vi "LiDARSteering.vi"() -> ()   [LabVIEW 2024]
uses:
  e33ea129-5426-40bd-9da2-e127971607b1.vi
  <vilib>/Instr/_visa.llb/VISA Configure Serial Port (Instr).vi
  <vilib>/Python/Open Venv Python Session.vi
  <vilib>/Instr/_visa.llb/VISA Set IO Buffer Mask.ctl
  <vilib>/Instr/_visa.llb/VISA Flush IO Buffer Mask.ctl
panel:
  out "inputsteer":dbl format="%#_13g"
  in  "HENES":refnum<visa-resource-name>="COM3"
  out "E-STOP":bool
  out "Remote_M/A":bool
  out "Steer_Feed":dbl
  out "Alive_PCU":u8(slide) scale=0.0..254.0
  out "Gear_Feed":u8
  out "Speed_Feed(RPM)":dbl format="%#_g rpm"
  out "버퍼 읽기":string
  out "Speed_Feed(m/s)":dbl
  in  "HLV_Gear 2":u8
  in  "HLV_A/M":bool=TRUE
  in  "HLV_E-stop":bool
  out "버퍼 쓰기":string
  in  "InputSpeed":i16
  out "HENES Loop Time":u32=20
  out "Input_Spd(cmd)":dbl=538.4742241275792
  in  "GoBack":bool
  in  "InputSteer(cmd)":dbl=28.559259641865033
  in  "HLV_Gear":u8
  out "PointCloud":T1(graph)=[{"appended array"=[700.0, 700.0, 3500.0, 3500.0, -3500.0, -3500.0, -700.0, -700.0, 700.0], "appended array"=[800.0, -800.0, -800.0, 5200.0, 5200.0, -800.0, -800.0, 800.0, 800.0]}, {"appended array"=[-450.0], "appended array"=[-250.0]}, {"appended array"=[-450.0, -450.0, -800.0, -800.0, 0.0, 0.0, -450.0], "appended array"=[100.0, -800.0, -800.0, 1200.0, 1200.0, 100.0, 100.0]}, {"appended array"=[800.0, 750.0, 800.0, 800.0, 800.0, 800.0, 800.0], "appended array"=[400.0, 350.0, 350.0, 300.0, 250.0, 200.0, 150.0]}, {"appended array"=[450.0, 450.0, 800.0, 800.0, 0.0, 0.0, 450.0], "appended array"=[100.0, -800.0, -800.0, 1200.0, 1200.0, 100.0, 100.0]}, {"appended array"=array[442 elements], "appended array"=array[442 elements]}, {"appended array"=[4.2861222383783204e-13, 0.0], "appended array"=[7000.0, 0.0]}, {"appended array"=[500.0, 500.0, -500.0, -500.0, 500.0], "appended array"=[100.0, 950.0, 950.0, 100.0, 100.0]}]
  in  "격자크기":dbl=50.0
  out "LidarLoop":u32=101
  in  "Ratio_Threshold":i32=4
  in  "min_samples":i32=2
  in  "eps":i32=100
  in  "Spacing":i32=100
  in  "Threshold":i32=2100
  in  "Looking Y":i32=5200
  in  "Looking X":i32=3500
  out "Anthena_Steer":i32
  out "NearSteer":dbl=28.559259641865033
  out "TooClose":bool=TRUE
  out "PythonLoop":u32=101
  in  "LiDAR":refnum<visa-resource-name>="COM5"
  out "VEstop":bool
  in  "length":dbl=1300.0
  out "read buffer":string
  out "Clustering Error":errorcluster
  out "GobackROI":cluster{i32[], i32[]}={[500, 500, -500, -500, 500], [100, 950, 950, 100, 100]}
  in  "Stop":bool
  out "TargetDerection":cluster{dbl[], dbl[]}={[4.2861222383783204e-13, 0.0], [7000.0, 0.0]}
  out "Y_arraysREAL":i32[](array[numeric])=[1650, 1650, 1650, 1650, 1650, 1650, 1650, 1650, 1700, 1700, 1700, 1700, 1700, 1700, 1700, 1700, 1700, 1700, 1700, 1750, 1700]
  out "X_arraysREAL":i32[](array[numeric])=[1000, 1050, 1100, 1150, 1200, 1250, 1300, 1350, 1350, 1400, 1450, 1500, 1550, 1600, 1650, 1700, 1750, 1800, 1850, 1850, 1900]
  out "LookingAt":cluster{i32[], i32[]}={[700, 700, 3500, 3500, -3500, -3500, -700, -700, 700], [800, -800, -800, 5200, 5200, -800, -800, 800, 800]}
  out "NearCarPointsRight":cluster{"ROI_IN_X":dbl[], "ROI_IN_Y":dbl[]}={"ROI_IN_X"=[750.0, 800.0, 800.0, 800.0, 800.0, 800.0], "ROI_IN_Y"=[350.0, 350.0, 300.0, 250.0, 200.0, 150.0]}
  out "NearCarROIRight":cluster{i32[], i32[]}={[450, 450, 800, 800, 0, 0, 450], [100, -800, -800, 1200, 1200, 100, 100]}
  out "Clustered":T2
  out "NearCarROILeft":cluster{i32[], i32[]}={[-450, -450, -800, -800, 0, 0, -450], [100, -800, -800, 1200, 1200, 100, 100]}
  out "NearCarPointsLeft":cluster{"ROI_IN_X":dbl[], "ROI_IN_Y":dbl[]}={"ROI_IN_X"=[-450.0, -550.0], "ROI_IN_Y"=[-250.0, -300.0]}
  out "Y_arrays":dbl[](array[numeric])=[1650.0, 1650.0, 1650.0, 1650.0, 1650.0, 1650.0, 1650.0, 1700.0, 1700.0, 1700.0, 1700.0, 1700.0, 1700.0, 1700.0, 1700.0, 1700.0, 1700.0, 1700.0, 1750.0, 1700.0, 1700.0, 1750.0, 1750.0, 1750.0, 1750.0, 1750.0, 1750.0, 1750.0, 1750.0, 1750.0, 1750.0, 1750.0, 1800.0, 1800.0, 1800.0, 1800.0, 1800.0, 1800.0, 1800.0, 1800.0, 1800.0, 1800.0, 1800.0, 1800.0, 1800.0, 1800.0, 1800.0, 1800.0, 1800.0, 1850.0, 1850.0, 1850.0, 350.0, 350.0, 350.0, 300.0, 250.0, 200.0, 200.0, 150.0, 150.0, 100.0, 50.0, 0.0, -50.0, -100.0, -150.0, -200.0, -250.0, -300.0, -300.0, -350.0, -400.0, -450.0, -500.0, -550.0, -600.0, -650.0, -700.0, -750.0, -800.0, -800.0, -750.0, -750.0, -700.0, -700.0, -650.0, -600.0, -550.0, -550.0, -500.0, -450.0, -400.0, -350.0, -300.0, -250.0, -200.0, -150.0, -100.0, -50.0, 0.0, 50.0, 100.0, 150.0, 200.0, 250.0, 300.0, 350.0, 400.0, 400.0, 450.0, 500.0, 550.0, 600.0, 600.0, 650.0, 650.0, 700.0, 700.0, 750.0, 750.0, 800.0, 800.0, 850.0, 850.0, 900.0, 900.0, 950.0, 950.0, 1000.0, 1000.0, 1050.0, 1050.0, 1100.0, 1100.0, 1150.0, 1150.0, 1200.0, 1200.0, 1250.0, 1250.0, 1300.0, 1300.0, 1350.0, 1400.0, 1450.0, 1500.0, 1550.0, 1600.0, 1650.0, 1700.0, 1750.0, 1800.0, 1850.0, 1900.0, 1950.0, 2000.0, 2050.0, 2100.0, 2150.0, 2200.0, 2250.0, 2300.0, 2350.0, 2400.0, 2450.0, 2500.0, 2550.0, 2600.0, 2600.0, 2650.0, 2700.0, 2750.0, 2800.0, 2850.0, 2900.0, 2950.0, 3000.0, 3050.0, 3100.0, 3150.0, 3200.0, 3250.0, 3300.0, 3350.0, 3400.0, 3450.0, 3450.0, 3500.0, 3550.0, 3600.0, 3650.0, 3700.0, 3750.0, 3800.0, 3850.0, 3900.0, 3950.0, 4000.0, 4000.0, 4100.0, 4150.0, 4200.0, 4250.0, 4300.0, 4350.0, 4400.0, 4450.0, 4500.0, 4550.0, 4600.0, 4650.0, 4700.0, 4750.0, 4800.0, 4900.0, 4950.0, 5000.0, 5050.0, 5100.0, 5150.0, 4500.0, 4500.0, 4600.0, 4550.0, 3800.0, 3700.0, 3650.0, 3600.0, 3550.0, 3500.0, 3500.0, 3450.0, 3400.0, 3350.0, 3300.0, 3250.0, 3250.0, 3200.0, 3150.0, 3200.0, 3200.0, 3200.0, 3400.0, 3450.0, 3200.0, 4700.0, 4700.0, 3700.0, 3450.0, 3400.0, 3450.0, 3500.0, 3500.0, 3450.0, 3400.0, 3400.0, 3350.0, 3300.0, 3300.0, 3250.0, 1600.0, 1600.0, 1650.0, 1600.0, 1650.0, 1735.0877192982457, -160.3448275862069, 1825.7462686567164, 5025.0, 4500.0, 4575.0, 3392.1052631578946, 3425.0, 4700.0, 3395.8333333333335, 1827.3513645224173, 1919.6150097465888, 2011.8786549707602, 2104.142300194932, 2196.4059454191033, 2288.669590643275, 2380.9332358674465, 2473.196881091618, 2565.4605263157896, 2657.7241715399614, 2749.9878167641327, 2842.251461988304, 2934.5151072124754, 3026.778752436647, 3119.042397660819, 3211.3060428849903, 3303.5696881091617, 1824.0304709141276, 1912.9732225300093, 2001.9159741458911, 2090.858725761773, 2179.801477377655, 2268.7442289935366, 2357.6869806094182, 2446.6297322253004, 2535.572483841182, 2624.5152354570637, 2713.457987072946, 2802.400738688827, 2891.343490304709, 2980.2862419205912, 3069.228993536473, 3158.1717451523546, 3247.114496768236, 3336.057248384118, 1817.938596491228, 1900.7894736842106, 1983.640350877193, 2066.4912280701756, 2149.342105263158, 2232.1929824561403, 2315.043859649123, 2397.8947368421054, 2480.745614035088, 2563.59649122807, 2646.4473684210525, 2729.2982456140353, 2812.149122807017, 2895.0, 2977.8508771929824, 3060.7017543859647, 3143.5526315789475, 3226.4035087719294, 3309.254385964912, 4515.0, 4530.0, 4545.0, 4560.0, 4407.675438596491, 4315.350877192983, 4223.026315789473, 4130.701754385965, 4038.377192982456, 3946.0526315789475, 3853.7280701754385, 3761.40350877193, 3669.078947368421, 3576.754385964912, 3484.4298245614036, 4417.307692307692, 4334.615384615385, 4251.923076923077, 4169.2307692307695, 4086.5384615384614, 4003.846153846154, 3921.153846153846, 3838.4615384615386, 3755.769230769231, 3673.076923076923, 3590.3846153846152, 3507.6923076923076, 4588.888888888889, 4602.777777777777, 4616.666666666667, 4630.555555555556, 4644.444444444444, 4658.333333333333, 4672.222222222223, 4686.111111111111, 4479.166666666667, 4383.333333333333, 4287.5, 4191.666666666667, 4095.8333333333335, 4000.0, 3904.166666666667, 3808.3333333333335, 3712.5, 3616.666666666667, 3520.8333333333335, 3403.0701754385964, 3414.035087719298, 3392.6378446115286, 3393.1704260651627, 3393.7030075187968, 3394.2355889724313, 3394.7681704260654, 3395.3007518796994, 3417.7083333333335, 3410.416666666667, 3403.125, 4684.615384615385, 4669.2307692307695, 4653.846153846154, 4638.461538461538, 4623.076923076923, 4607.692307692308, 4592.307692307692, 4576.923076923077, 4561.538461538462, 4546.153846153846, 4530.7692307692305, 4515.384615384615, 4606.8452380952385, 4513.690476190476, 4420.535714285715, 4327.380952380952, 4234.226190476191, 4141.071428571428, 4047.916666666667, 3954.761904761905, 3861.607142857143, 3768.452380952381, 3675.2976190476193, 3582.1428571428573, 3488.9880952380954, 3486.538461538462, 3577.24358974359, 3667.9487179487182, 3758.653846153846, 3849.3589743589746, 3940.0641025641025, 4030.769230769231, 4121.474358974359, 4212.179487179487, 4302.884615384615, 4393.589743589744, 4484.294871794872]
  out "X_arrays":dbl[](array[numeric])=[1050.0, 1100.0, 1150.0, 1200.0, 1250.0, 1300.0, 1350.0, 1350.0, 1400.0, 1450.0, 1500.0, 1550.0, 1600.0, 1650.0, 1700.0, 1750.0, 1800.0, 1850.0, 1850.0, 1900.0, 1950.0, 2000.0, 2050.0, 2100.0, 2150.0, 2200.0, 2250.0, 2300.0, 2350.0, 2400.0, 2450.0, 2500.0, 2500.0, 2550.0, 2600.0, 2650.0, 2700.0, 2750.0, 2800.0, 2850.0, 2900.0, 2950.0, 3000.0, 3050.0, 3100.0, 3150.0, 3200.0, 3250.0, 3300.0, 3350.0, 3400.0, 3450.0, 750.0, 800.0, 850.0, 800.0, 800.0, 800.0, 850.0, 800.0, 850.0, 850.0, 850.0, 850.0, 850.0, 850.0, 850.0, 850.0, 850.0, 850.0, 900.0, 900.0, 900.0, 900.0, 900.0, 900.0, 900.0, 900.0, 900.0, 900.0, 900.0, -2250.0, -2250.0, -2300.0, -2300.0, -2250.0, -2300.0, -2300.0, -2300.0, -2350.0, -2300.0, -2300.0, -2300.0, -2300.0, -2300.0, -2300.0, -2300.0, -2300.0, -2300.0, -2300.0, -2300.0, -2300.0, -2300.0, -2300.0, -2300.0, -2300.0, -2300.0, -2300.0, -2250.0, -2300.0, -2300.0, -2300.0, -2300.0, -2300.0, -2250.0, -2250.0, -2300.0, -2250.0, -2300.0, -2300.0, -2250.0, -2300.0, -2250.0, -2300.0, -2250.0, -2300.0, -2250.0, -2250.0, -2300.0, -2300.0, -2250.0, -2250.0, -2300.0, -2250.0, -2300.0, -2250.0, -2300.0, -2250.0, -2300.0, -2300.0, -2250.0, -2300.0, -2250.0, -2250.0, -2250.0, -2250.0, -2250.0, -2250.0, -2250.0, -2250.0, -2250.0, -2250.0, -2250.0, -2250.0, -2250.0, -2250.0, -2250.0, -2250.0, -2250.0, -2250.0, -2250.0, -2250.0, -2250.0, -2250.0, -2250.0, -2250.0, -2250.0, -2250.0, -2250.0, -2300.0, -2300.0, -2300.0, -2300.0, -2300.0, -2300.0, -2300.0, -2300.0, -2300.0, -2300.0, -2300.0, -2300.0, -2300.0, -2300.0, -2300.0, -2300.0, -2300.0, -2300.0, -2350.0, -2350.0, -2350.0, -2350.0, -2350.0, -2350.0, -2350.0, -2350.0, -2350.0, -2350.0, -2350.0, -2350.0, -2400.0, -2400.0, -2400.0, -2400.0, -2400.0, -2400.0, -2400.0, -2400.0, -2400.0, -2400.0, -2400.0, -2400.0, -2400.0, -2400.0, -2400.0, -2400.0, -2450.0, -2450.0, -2450.0, -2450.0, -2450.0, -2450.0, 650.0, 700.0, 1100.0, 1150.0, 950.0, 950.0, 950.0, 950.0, 950.0, 950.0, 1000.0, 1000.0, 1000.0, 1000.0, 1000.0, 1000.0, 1050.0, 1050.0, 1050.0, 1100.0, 1150.0, 1200.0, 1300.0, 1350.0, 1250.0, 1900.0, 1950.0, 1600.0, 1500.0, 1550.0, 1600.0, 1600.0, 1650.0, 1650.0, 1650.0, 1700.0, 1650.0, 1650.0, 1700.0, 1700.0, 900.0, 950.0, 950.0, 1000.0, 1000.0, 2118.4210526315787, 856.8965517241379, -2300.0, -2450.0, 675.0, 1125.0, 1028.9473684210527, 1325.0, 1925.0, 1633.3333333333333, 2091.4717348927875, 2064.522417153996, 2037.5730994152045, 2010.623781676413, 1983.6744639376216, 1956.7251461988303, 1929.7758284600388, 1902.8265107212474, 1875.877192982456, 1848.9278752436646, 1821.9785575048732, 1795.029239766082, 1768.0799220272904, 1741.130604288499, 1714.1812865497075, 1687.231968810916, 1660.2826510721247, 2076.6620498614957, 2034.9030470914126, 1993.1440443213294, 1951.3850415512463, 1909.6260387811633, 1867.8670360110802, 1826.108033240997, 1784.349030470914, 1742.590027700831, 1700.8310249307478, 1659.0720221606648, 1617.3130193905818, 1575.5540166204987, 1533.7950138504154, 1492.0360110803324, 1450.2770083102494, 1408.5180055401663, 1366.759002770083, 2063.9473684210525, 2009.4736842105262, 1954.9999999999998, 1900.5263157894735, 1846.0526315789473, 1791.5789473684208, 1737.1052631578946, 1682.6315789473683, 1628.157894736842, 1573.6842105263158, 1519.2105263157894, 1464.736842105263, 1410.2631578947367, 1355.7894736842104, 1301.3157894736842, 1246.842105263158, 1192.3684210526317, 1137.8947368421054, 1083.421052631579, 765.0, 855.0, 945.0, 1035.0, 704.4956140350878, 733.9912280701755, 763.4868421052631, 792.9824561403509, 822.4780701754387, 851.9736842105264, 881.469298245614, 910.9649122807018, 940.4605263157896, 969.9561403508773, 999.4517543859649, 725.0, 775.0, 825.0, 875.0, 925.0, 975.0, 1025.0, 1075.0, 1125.0, 1175.0, 1225.0, 1275.0, 1213.888888888889, 1302.7777777777778, 1391.6666666666665, 1480.5555555555557, 1569.4444444444443, 1658.3333333333333, 1747.2222222222222, 1836.111111111111, 1141.6666666666667, 1158.3333333333333, 1175.0, 1191.6666666666667, 1208.3333333333333, 1225.0, 1241.6666666666667, 1258.3333333333333, 1275.0, 1291.6666666666667, 1308.3333333333333, 1127.6315789473686, 1226.3157894736842, 1115.2882205513786, 1201.6290726817042, 1287.96992481203, 1374.310776942356, 1460.6516290726815, 1546.9924812030074, 1402.0833333333333, 1479.1666666666665, 1556.25, 1828.8461538461538, 1732.6923076923076, 1636.5384615384614, 1540.3846153846152, 1444.2307692307693, 1348.076923076923, 1251.9230769230767, 1155.7692307692307, 1059.6153846153848, 963.4615384615385, 867.3076923076922, 771.1538461538462, 1904.1666666666667, 1883.3333333333333, 1862.5, 1841.6666666666667, 1820.8333333333333, 1800.0, 1779.1666666666665, 1758.3333333333333, 1737.5, 1716.6666666666665, 1695.8333333333333, 1675.0, 1654.1666666666665, 1594.230769230769, 1555.128205128205, 1516.0256410256409, 1476.923076923077, 1437.8205128205127, 1398.7179487179487, 1359.6153846153845, 1320.5128205128203, 1281.4102564102564, 1242.3076923076924, 1203.2051282051282, 1164.102564102564]
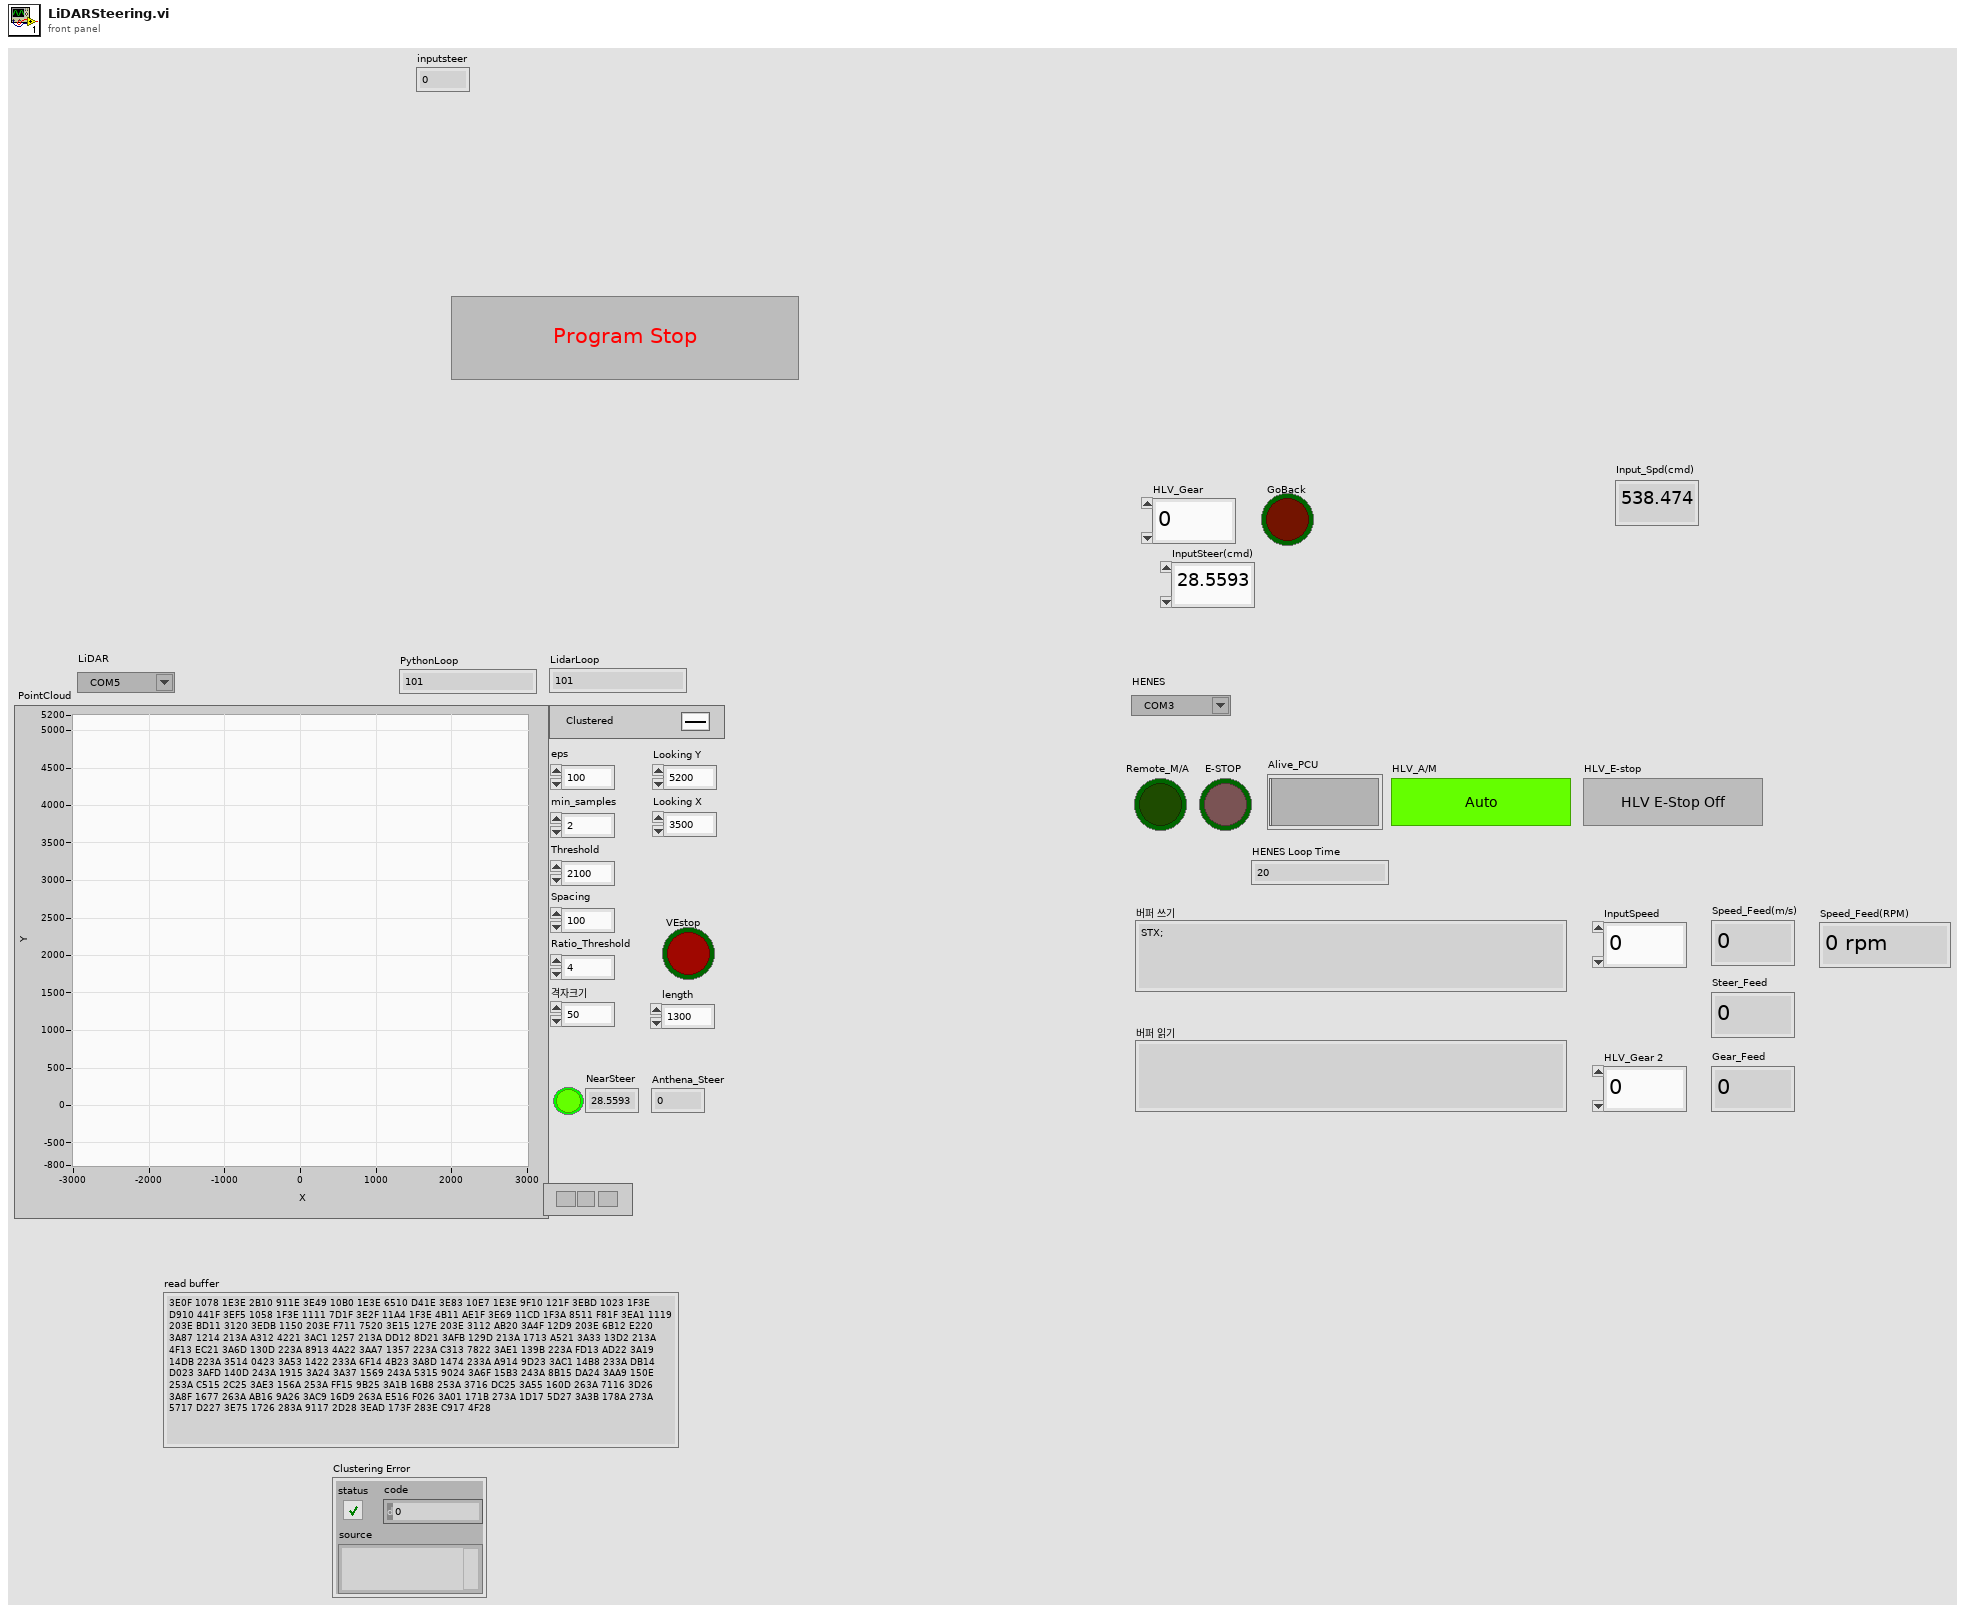
[diagram p1: front panel]
types:
  T1 = cluster{"appended array":dbl[], "appended array":dbl[]}[]
  T2 = cluster{"appended array":dbl[], "appended array":dbl[]}
  T3 = cluster{"HENES_M/A":u8, "HENES_E-Stop":u8, "HENES_Gear":u8, "HENES_Speed":i16, "HENES_Steer":i16, "HENES_Alive":u8}
  T4 = typedef "VISA Flush IO Buffer Mask.ctl" = u16
  T5 = typedef "VISA Set IO Buffer Mask.ctl" = u16
  T6 = cluster{"HLV_M/A_Status":u8, "HLV_E-Stop":u8, "HLV_Gear":u8, "HLV_Speed":i16, "HLV_Steer":i16, "HLV_Alive":u8}
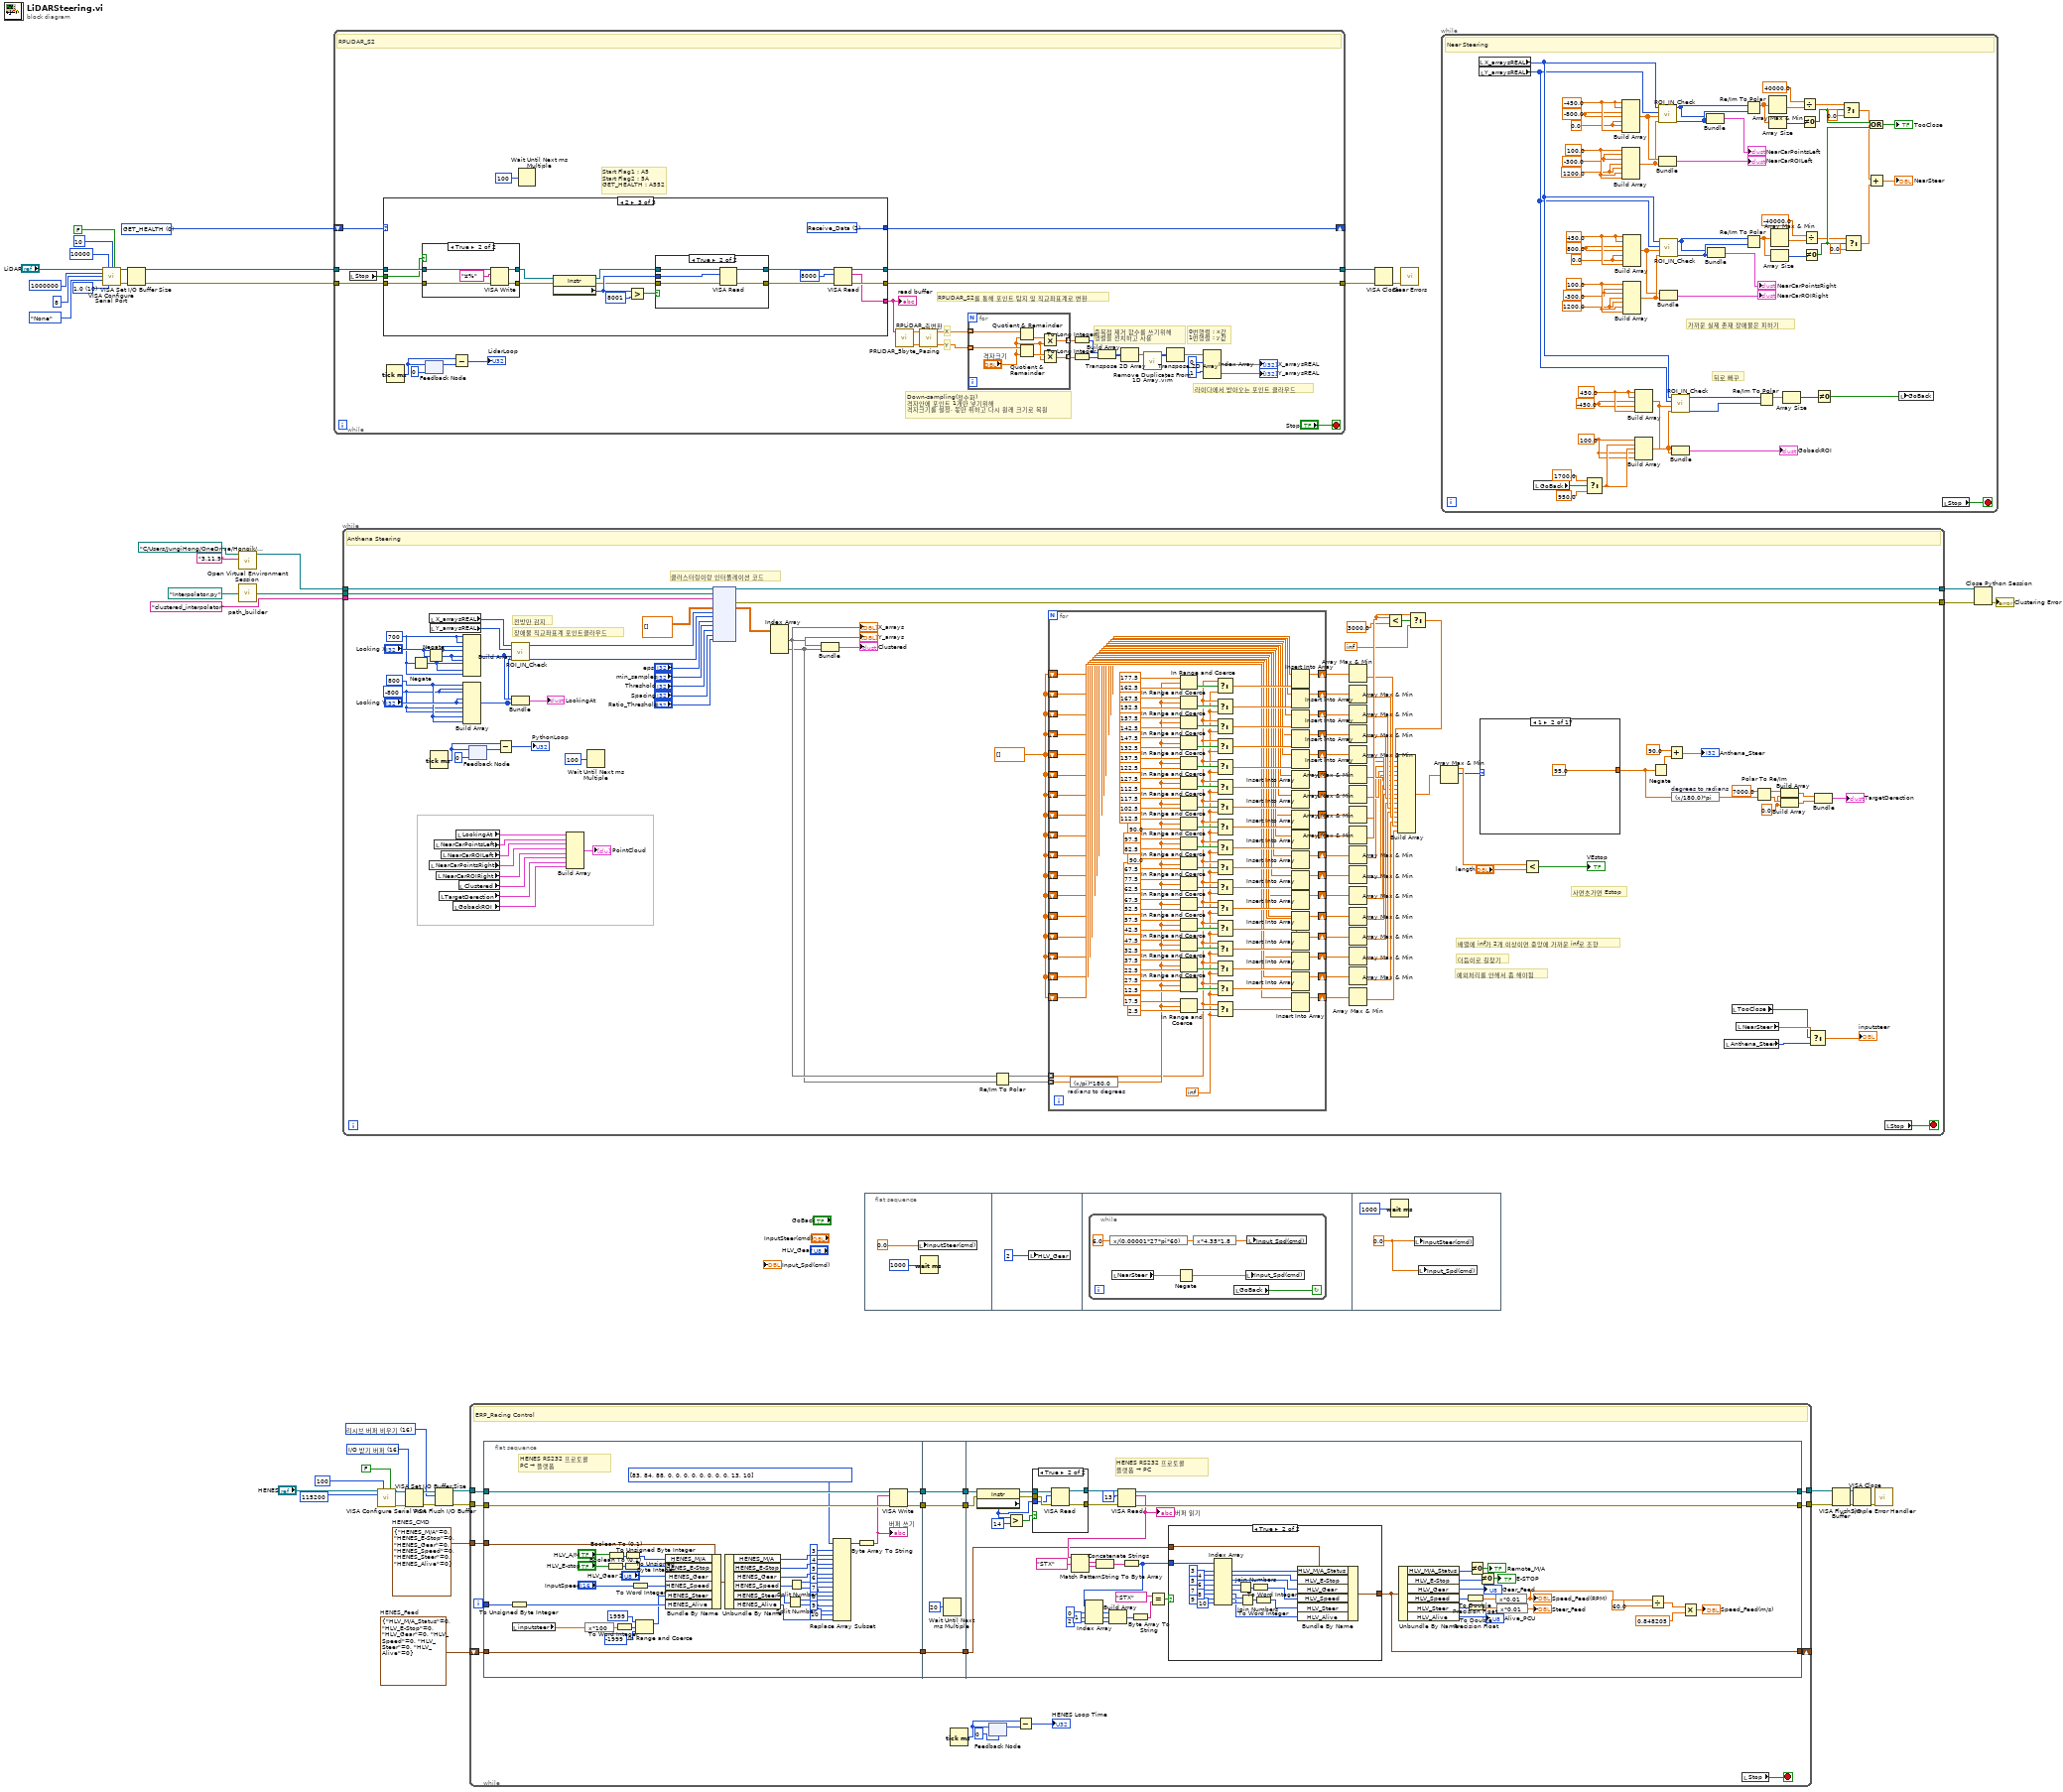
[diagram p0: block diagram]
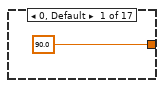
[diagram p4: hidden frame]
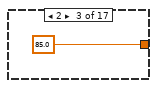
[diagram p5: hidden frame]
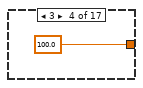
[diagram p6: hidden frame]
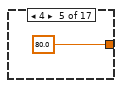
[diagram p7: hidden frame]
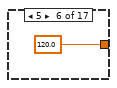
[diagram p8: hidden frame]
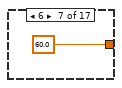
[diagram p9: hidden frame]
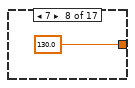
[diagram p10: hidden frame]
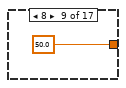
[diagram p11: hidden frame]
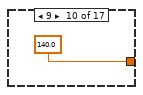
[diagram p12: hidden frame]
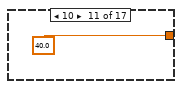
[diagram p13: hidden frame]
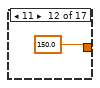
[diagram p14: hidden frame]
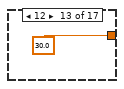
[diagram p15: hidden frame]
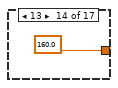
[diagram p16: hidden frame]
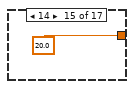
[diagram p17: hidden frame]
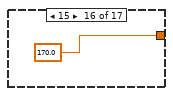
[diagram p18: hidden frame]
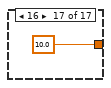
[diagram p19: hidden frame]
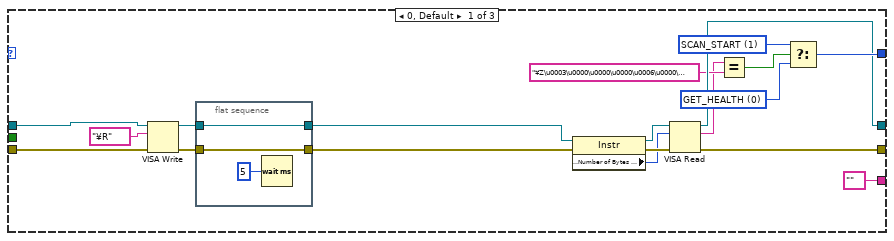
[diagram p20: hidden frame]
diagram:
  w2 = T3 {"HENES_M/A"=0, "HENES_E-Stop"=0, "HENES_Gear"=0, "HENES_Speed"=0, "HENES_Steer"=0, "HENES_Alive"=0}  # HENES_CMD
  w5 = T4 16 items=["리시브 버퍼 비우기"=16, "전달 버퍼 디바이스에 쓰기"=32, "리시브 버퍼 비우기(I/O 없음)"=64, "전달 버퍼 비우기"=128] ("Mask")
  w8 = T5 16 items=["I/O 받기 버퍼"=16, "I/O 전달 버퍼"=32, "I/O 받기와 전달 버퍼"=48] ("Mask")
  w12 = T6 {"HLV_M/A_Status"=0, "HLV_E-Stop"=0, "HLV_Gear"=0, "HLV_Speed"=0, "HLV_Steer"=0, "HLV_Alive"=0}  # HENES_Feed
  w30 = u16 10 items=["1.0"=10, "1.5"=15, "2.0"=20] ("stop bits (10: 1 bit)")
  w32 = u16 0 items=["GET_HEALTH", "SCAN_START", "Receive_Data"]
  n1 = call-poly "VISA Configure Serial Port"("VISA resource name"="LiDAR", "timeout (10sec)"=u32 10000, "termination char\n(0xA = '\\n' = LF)"=u8 10 ("termination char\n(0xA = '\\n' = LF)"), "Enable Termination\nChar (T)"=FALSE ("Enable Termination\nChar (T)"), "baud rate (9600)"=u32 1000000, "data bits (8)"=u16 8, "parity (0:none)"=enum16{"None", "Odd", "Even", "Mark", "Space"}."None", "stop bits (10: 1 bit)"=w30) -> ("VISA resource name out"=w39:refnum<visa-resource-name>, "error out"=w38:errorcluster)  [unwired: 6 in]
  n2 = VISA Set I/O Buffer Size(VISA resource name=w39, error in (no error)=w38) -> (VISA resource name out=w34:refnum<visa-resource-name>, error out=w33:errorcluster)  [unwired: 2 in]
  n3 = call-poly <vilib>:"Open Virtual Environment Session.vi"("Python version"="3.11.9", "Env path"=path "C:/Users/JungiHong/OneDrive/Hongik/HI-RACE/2026-01/.venv" ("Name")) -> ("session out"=w21:refnum<k35>)  [unwired: 8 in, 1 out]
  n4 = call "path_builder.vi"("Name"=path "Interpolator.py") -> ("appended path"=w25:path)
  n5 = while {
    tunnel: [w64] -> w43
    tunnel: [w65] -> w42
    tunnel: w34 -> [w73]
    tunnel: w33 -> [w72]
    shift-right: [w71] -> _
    shift-left: w32 -> [w74]
    stop <- "Stop" stop-if-true
    # "라이다에서 받아오는 포인트 클라우드"
    # "RPLIDAR_S2를 통해 포인트 탐지 및 직교좌표계로 변환"
    # "Start Flag1 : A5\nStart Flag2 : 5A \nGET_HEALTH : A552"
    # "0번행렬 : x값\n1번행렬 : y값"
    # "중복점 제거 함수를 쓰기위해\n행렬을 전치하고 사용"
    # "Down-sampling(정수화)\n격자안에 포인트 1개만 넣기위해\n격자크기를 설정, 몫만 취하고 다시 원래 크기로 복원"
    # "Y"
    # "X"
    # "RPLIDAR_S2"
    n6 = local read "Stop"() -> (w70:bool)
    n7 = case shown="2" w74 {
      tunnel: w73 -> [w99 w117 w140]
      tunnel: w72 -> [w98 w116 w139]
      tunnel: [w100 w113 w126] -> w71
      tunnel: [w89 w114 w142] -> w65
      tunnel: [w88 w115 w141] -> w64
      tunnel: w70 -> [_ _ w138]
      tunnel: ["" ("read buffer") w111 w137] -> w49
      frame 0, Default {
        w82 = u16 0 items=["GET_HEALTH", "SCAN_START", "Receive_Data"]
        w83 = u16 1 items=["GET_HEALTH", "SCAN_START", "Receive_Data"]
        n8 = VISA Write(VISA resource name=w99, write buffer="¥R", error in (no error)=w98) -> (VISA resource name out=w93:refnum<visa-resource-name>, error out=w92:errorcluster)  [unwired: 1 out]
        n9 = flat-sequence {
          tunnel: w93 -> [w102]
          tunnel: w92 -> [w101]
          tunnel: [w102] -> w91
          tunnel: [w101] -> w90
          frame #0 {
            n10 = Wait (ms)(milliseconds to wait=u32 5 ("대기 시간 (ms)")) -> ()  [unwired: 1 out]
          }
        }
        n11 = property class="Instr"(reference=w91, error in=w90) -> (reference out=w96:refnum<visa-resource-name>, error out=w95:errorcluster, "Serial Settings:Number of Bytes at Serial Port"=w94:u32)
        n12 = VISA Read(VISA resource name=w96, byte count=w94, error in (no error)=w95) -> (VISA resource name out=w88:refnum<visa-resource-name>, read buffer=w85:string, error out=w89:errorcluster)  [unwired: 1 out]
        n13 = Equal?(x=w85, y="¥Z\u0003\u0000\u0000\u0000\u0006\u0000\u0000\u0000") -> (x = y?=w86:bool)
        n14 = Select(t=w83, s=w86, f=w82) -> (s? t:f=w100:u16)
      }
      frame 1 {
        w104 = u16 2 items=["GET_HEALTH", "SCAN_START", "Receive_Data"]
        w105 = u16 1 items=["GET_HEALTH", "SCAN_START", "Receive_Data"]
        w118 = "¥Z\u0005\u0000\u0000@"
        n15 = VISA Write(VISA resource name=w117, write buffer="¥ \u0000", error in (no error)=w116) -> (VISA resource name out=w120:refnum<visa-resource-name>, error out=w121:errorcluster)  [unwired: 1 out]
        n16 = flat-sequence {
          tunnel: w120 -> [w124]
          tunnel: w121 -> [w123]
          tunnel: [w124] -> w107
          tunnel: [w123] -> w106
          frame #0 {
            n17 = Wait (ms)(milliseconds to wait=u32 5 ("대기 시간 (ms)")) -> ()  [unwired: 1 out]
          }
        }
        n18 = property class="Instr"(reference=w107, error in=w106) -> (reference out=w110:refnum<visa-resource-name>, error out=w109:errorcluster, "Serial Settings:Number of Bytes at Serial Port"=w108:u32)
        n19 = VISA Read(VISA resource name=w110, byte count=w108, error in (no error)=w109) -> (VISA resource name out=w115:refnum<visa-resource-name>, read buffer=w111:string, error out=w114:errorcluster)  [unwired: 1 out]
        n20 = Match Pattern(string=w111, regular expression=w118) -> (match substring=w112:string)  [unwired: 1 in, 3 out]
        n21 = Equal?(x=w112, y=w118) -> (x = y?=w122:bool)
        n22 = Select(t=w104, s=w122, f=w105) -> (s? t:f=w113:u16)
      }
      frame 2 {
        w126 = u16 2 items=["GET_HEALTH", "SCAN_START", "Receive_Data"]
        n23 = case shown="True" w138 {
          tunnel: w140 -> [w151 w155]
          tunnel: w139 -> [w150 w154]
          tunnel: [w151 w153] -> w136
          tunnel: [w150 w152] -> w135
          frame False {
          }
          frame True {
            n24 = VISA Write(VISA resource name=w155, write buffer="¥%", error in (no error)=w154) -> (VISA resource name out=w153:refnum<visa-resource-name>, error out=w152:errorcluster)  [unwired: 1 out]
          }
        }
        n25 = property class="Instr"(reference=w136, error in=w135) -> (reference out=w131:refnum<visa-resource-name>, error out=w130:errorcluster, "Serial Settings:Number of Bytes at Serial Port"=w132:u32)
        n26 = Greater?(x=w132, y=u32 8001) -> (0:w134:bool)
        n27 = case shown="True" w134 {
          tunnel: w131 -> [w144 w149]
          tunnel: w132 -> [_ w148]
          tunnel: w130 -> [w143 w147]
          tunnel: [w144 w146] -> w129
          tunnel: [w143 w145] -> w128
          frame False {
          }
          frame True {
            n28 = VISA Read(VISA resource name=w149, byte count=w148, error in (no error)=w147) -> (VISA resource name out=w146:refnum<visa-resource-name>, error out=w145:errorcluster)  [unwired: 2 out]
          }
        }
        n29 = VISA Read(VISA resource name=w129, byte count=u32 8000, error in (no error)=w128) -> (VISA resource name out=w141:refnum<visa-resource-name>, read buffer=w137:string, error out=w142:errorcluster)  [unwired: 1 out]
      }
    }
    "read buffer" <- w49
    n30 = Tick Count (ms)() -> (millisecond timer value=w69:u32)
    n31 = feedback #1(u32 0 ("millisecond timer value")) -> (w68:u32)
    n32 = feedback-in #1(w69) -> ()
    n33 = Subtract(x=w69, y=w68) -> (x-y=→"LidarLoop":u32)
    n34 = Wait Until Next ms Multiple(millisecond multiple=u32 100) -> ()  [unwired: 1 out]
    n35 = call "PRLIDAR_5byte_Pasing.vi"("RPLIDAR_Data"=w49) -> ("Theta(deg)"=w52:dbl[], "Distance(mm)"=w53:dbl[])  [unwired: 9 in]
    n36 = call "RPLiDAR_축변환.vi"("Theta(deg)"=w52, "Distance(mm)"=w53) -> ("Y"=w50:dbl[], "X"=w51:dbl[])  [unwired: 8 in]
    n37 = for {
      tunnel: w51 -> [w81] mode=indexing
      tunnel: w50 -> [w80] mode=indexing
      tunnel: [w77] -> w62 mode=indexing
      tunnel: [w76] -> w63 mode=indexing
      n38 = Quotient & Remainder(x=w81, y="격자크기") -> (floor(x/y)=w79:dbl)  [unwired: 1 out]
      n39 = Quotient & Remainder(x=w80, y="격자크기") -> (floor(x/y)=w78:dbl)  [unwired: 1 out]
      n40 = Multiply(x=w79, y="격자크기") -> (x*y=w77:dbl)
      n41 = Multiply(x=w78, y="격자크기") -> (x*y=w76:dbl)
    }
    n42 = To Long Integer(number=w62) -> (32bit integer=w57:i32[])
    n43 = To Long Integer(number=w63) -> (32bit integer=w56:i32[])
    n44 = Build Array(w57, w56) -> (w58:i32[][])
    n45 = Transpose 2D Array(2D array=w58) -> (transposed array=w54:i32[][])
    n46 = call "Remove Duplicates From 1D Array.vim"("array"=w54) -> ("array with duplicates removed"=w55:i32[][])  [unwired: 10 in]
    n47 = Transpose 2D Array(2D array=w55) -> (transposed array=w59:i32[][])
    n48 = Index Array(array=w59, index (row) #1=0 ("index (row)"), index (row) #2=1 ("index (row)")) -> (element #1=→"X_arraysREAL":i32[], element #2=→"Y_arraysREAL":i32[])  [unwired: 2 in]
  }
  n49 = while {
    tunnel: [w262] -> w29
    tunnel: "clustered_interpolator" ("function name") -> [w260]
    tunnel: w25 -> [w259]
    tunnel: w21 -> [w258]
    tunnel: [w261] -> w28
    stop <- w170 stop-if-true
    w173 = dbl[] []
    w175 = 0.0 ("r")
    w235 = -800
    w236 = 800
    w237 = 700
    # "사면초가면 Estop"
    # "배열에 inf가 2개 이상이면 중앙에 가까운 inf로 조향"
    # "예외처리를 안해서 좀 해야됨"
    # "더듬이로 길찾기"
    # "전방만 감지"
    # "장애물 직교좌표계 포인트클라우드"
    # "클러스터링이랑 인터폴레이션 코드"
    # "Anthena Steering"
    n50 = Negate(x=w237) -> (-x=w240:i32)
    n51 = Negate(x="Looking X") -> (-x=w241:i32)
    n52 = local read "X_arraysREAL"() -> (w234:i32[])
    n53 = local read "NearCarPointsRight"() -> (w167:cluster{"ROI_IN_X":dbl[], "ROI_IN_Y":dbl[]})
    n54 = local read "Y_arraysREAL"() -> (w233:i32[])
    n55 = Tick Count (ms)() -> (millisecond timer value=w245:u32)
    n56 = local read "NearCarPointsLeft"() -> (w164:cluster{"ROI_IN_X":dbl[], "ROI_IN_Y":dbl[]})
    n57 = local read "NearCarROIRight"() -> (w168:cluster{i32[], i32[]})
    n58 = local read "TargetDerection"() -> (w162:cluster{dbl[], dbl[]})
    n59 = local read "NearCarROILeft"() -> (w165:cluster{i32[], i32[]})
    n60 = local read "GobackROI"() -> (w161:cluster{i32[], i32[]})
    n61 = local read "LookingAt"() -> (w163:cluster{i32[], i32[]})
    n62 = local read "Clustered"() -> (w169:T2)
    n63 = Build Array(w237, w237, "Looking X", "Looking X", w241, w241, w240, w240, w237) -> (w243:i32[])
    n64 = Build Array(w236, w235, w235, "Looking Y", "Looking Y", w235, w235, w236, w236) -> (w242:i32[])
    n65 = feedback #2(u32 0 ("millisecond timer value")) -> (w246:u32)
    n66 = feedback-in #2(w245) -> ()
    n67 = Subtract(x=w245, y=w246) -> (x-y=→"PythonLoop":u32)
    n68 = call "ROI_IN_Check.vi"("도형Y좌표"=w242, "도형X좌표"=w243, "LiDAR_Y"=w233, "LiDAR_X"=w234) -> ("ROI_IN_Y"=w231:i32[], "ROI_IN_X"=w232:i32[])  [unwired: 6 in]
    n69 = Bundle(w243, w242) -> (→"LookingAt":cluster{i32[], i32[]})  [unwired: 1 in]
    n70 = Build Array(w163, w164, w165, w167, w168, w169, w162, w161) -> (→"PointCloud":T1)
    n71 = Wait Until Next ms Multiple(millisecond multiple=u32 100) -> ()  [unwired: 1 out]
    n72 = node(w258, w259, w260, dbl[][] [] ("appended array"), w232, w231, "eps", "min_samples", "Threshold", "Spacing", "Ratio_Threshold") -> (w261:refnum<k35>, w262:errorcluster, w257:dbl[][])  [unwired: 8 in, 2 out]
    n73 = Index Array(array=w257) -> (element #1=w172:dbl[], element #2=w171:dbl[])  [unwired: 4 in]
    "X_arrays" <- w172
    "Y_arrays" <- w171
    n74 = Bundle("appended array"=w172, "appended array"=w171) -> (→"Clustered":T2)  [unwired: 1 in]
    n75 = Re/Im To Polar(2:w171, 3:w172) -> (0:w179:dbl[], 1:w180:dbl[])
    n76 = for {
      tunnel: w179 -> [w385] mode=indexing
      tunnel: w180 -> [w307] mode=indexing
      shift-right: [w352] -> w181
      shift-left: w173 -> [w284]
      shift-right: [w351] -> w182
      shift-left: w173 -> [w285]
      shift-right: [w350] -> w183
      shift-left: w173 -> [w286]
      shift-right: [w349] -> w184
      shift-left: w173 -> [w287]
      shift-right: [w348] -> w185
      shift-left: w173 -> [w288]
      shift-right: [w347] -> w186
      shift-left: w173 -> [w289]
      shift-right: [w346] -> w187
      shift-left: w173 -> [w290]
      shift-right: [w345] -> w188
      shift-left: w173 -> [w291]
      shift-right: [w341] -> w194
      shift-left: w173 -> [w292]
      shift-right: [w305] -> w209
      shift-left: w173 -> [w293]
      shift-right: [w304] -> w210
      shift-left: w173 -> [w294]
      shift-right: [w303] -> w211
      shift-left: w173 -> [w295]
      shift-right: [w302] -> w212
      shift-left: w173 -> [w296]
      shift-right: [w298] -> w216
      shift-left: w173 -> [w280]
      shift-right: [w299] -> w215
      shift-left: w173 -> [w281]
      shift-right: [w300] -> w214
      shift-left: w173 -> [w282]
      shift-right: [w301] -> w213
      shift-left: w173 -> [w283]
      w306 = inf
      n77 = expression code="(x/pi)*180.0" "radians to degrees"(w385) -> (w325:dbl)
      n78 = In Range and Coerce(upper limit=177.5, x=w325, lower limit=162.5) -> (In Range?=w312:bool)  [unwired: 1 out]
      n79 = In Range and Coerce(upper limit=167.5, x=w325, lower limit=152.5 ("upper limit")) -> (In Range?=w313:bool)  [unwired: 1 out]
      n80 = In Range and Coerce(upper limit=157.5 ("lower limit"), x=w325, lower limit=142.5 ("upper limit")) -> (In Range?=w314:bool)  [unwired: 1 out]
      n81 = In Range and Coerce(upper limit=147.5 ("lower limit"), x=w325, lower limit=132.5 ("upper limit")) -> (In Range?=w315:bool)  [unwired: 1 out]
      n82 = In Range and Coerce(upper limit=137.5, x=w325, lower limit=122.5) -> (In Range?=w366:bool)  [unwired: 1 out]
      n83 = In Range and Coerce(upper limit=127.5, x=w325, lower limit=112.5) -> (In Range?=w368:bool)  [unwired: 1 out]
      n84 = In Range and Coerce(upper limit=117.5, x=w325, lower limit=102.5) -> (In Range?=w364:bool)  [unwired: 1 out]
      n85 = In Range and Coerce(upper limit=112.5, x=w325, lower limit=90.0) -> (In Range?=w363:bool)  [unwired: 1 out]
      n86 = In Range and Coerce(upper limit=97.5, x=w325, lower limit=82.5) -> (In Range?=w362:bool)  [unwired: 1 out]
      n87 = In Range and Coerce(upper limit=90.0, x=w325, lower limit=67.5) -> (In Range?=w361:bool)  [unwired: 1 out]
      n88 = In Range and Coerce(upper limit=77.5, x=w325, lower limit=62.5) -> (In Range?=w360:bool)  [unwired: 1 out]
      n89 = In Range and Coerce(upper limit=67.5, x=w325, lower limit=52.5) -> (In Range?=w359:bool)  [unwired: 1 out]
      n90 = In Range and Coerce(upper limit=57.5, x=w325, lower limit=42.5) -> (In Range?=w344:bool)  [unwired: 1 out]
      n91 = In Range and Coerce(upper limit=47.5, x=w325, lower limit=32.5) -> (In Range?=w323:bool)  [unwired: 1 out]
      n92 = In Range and Coerce(upper limit=37.5, x=w325, lower limit=22.5) -> (In Range?=w322:bool)  [unwired: 1 out]
      n93 = In Range and Coerce(upper limit=27.5, x=w325, lower limit=12.5) -> (In Range?=w321:bool)  [unwired: 1 out]
      n94 = In Range and Coerce(upper limit=17.5, x=w325, lower limit=2.5) -> (In Range?=w320:bool)  [unwired: 1 out]
      n95 = Select(t=w307, s=w312, f=w306) -> (s? t:f=w311:dbl)
      n96 = Select(t=w307, s=w313, f=w306) -> (s? t:f=w310:dbl)
      n97 = Select(t=w307, s=w314, f=w306) -> (s? t:f=w309:dbl)
      n98 = Select(t=w307, s=w315, f=w306) -> (s? t:f=w308:dbl)
      n99 = Select(t=w307, s=w366, f=w306) -> (s? t:f=w365:dbl)
      n100 = Select(t=w307, s=w368, f=w306) -> (s? t:f=w367:dbl)
      n101 = Select(t=w307, s=w364, f=w306) -> (s? t:f=w353:dbl)
      n102 = Select(t=w307, s=w363, f=w306) -> (s? t:f=w354:dbl)
      n103 = Select(t=w307, s=w362, f=w306) -> (s? t:f=w355:dbl)
      n104 = Select(t=w307, s=w361, f=w306) -> (s? t:f=w356:dbl)
      n105 = Select(t=w307, s=w360, f=w306) -> (s? t:f=w357:dbl)
      n106 = Select(t=w307, s=w359, f=w306) -> (s? t:f=w358:dbl)
      n107 = Select(t=w307, s=w344, f=w306) -> (s? t:f=w324:dbl)
      n108 = Select(t=w307, s=w323, f=w306) -> (s? t:f=w319:dbl)
      n109 = Select(t=w307, s=w322, f=w306) -> (s? t:f=w318:dbl)
      n110 = Select(t=w307, s=w321, f=w306) -> (s? t:f=w317:dbl)
      n111 = Select(t=w307, s=w320, f=w306) -> (s? t:f=w316:dbl)
      n112 = Insert Into Array(array=w280, new element=w311) -> (w298:dbl[])  [unwired: 1 in]
      n113 = Insert Into Array(array=w281, new element=w310) -> (w299:dbl[])  [unwired: 1 in]
      n114 = Insert Into Array(array=w282, new element=w309) -> (w300:dbl[])  [unwired: 1 in]
      n115 = Insert Into Array(array=w283, new element=w308) -> (w301:dbl[])  [unwired: 1 in]
      n116 = Insert Into Array(array=w284, new element=w365) -> (w352:dbl[])  [unwired: 1 in]
      n117 = Insert Into Array(array=w285, new element=w367) -> (w351:dbl[])  [unwired: 1 in]
      n118 = Insert Into Array(array=w286, new element=w353) -> (w350:dbl[])  [unwired: 1 in]
      n119 = Insert Into Array(array=w287, new element=w354) -> (w349:dbl[])  [unwired: 1 in]
      n120 = Insert Into Array(array=w288, new element=w355) -> (w348:dbl[])  [unwired: 1 in]
      n121 = Insert Into Array(array=w289, new element=w356) -> (w347:dbl[])  [unwired: 1 in]
      n122 = Insert Into Array(array=w290, new element=w357) -> (w346:dbl[])  [unwired: 1 in]
      n123 = Insert Into Array(array=w291, new element=w358) -> (w345:dbl[])  [unwired: 1 in]
      n124 = Insert Into Array(array=w292, new element=w324) -> (w341:dbl[])  [unwired: 1 in]
      n125 = Insert Into Array(array=w293, new element=w319) -> (w305:dbl[])  [unwired: 1 in]
      n126 = Insert Into Array(array=w294, new element=w318) -> (w304:dbl[])  [unwired: 1 in]
      n127 = Insert Into Array(array=w295, new element=w317) -> (w303:dbl[])  [unwired: 1 in]
      n128 = Insert Into Array(array=w296, new element=w316) -> (w302:dbl[])  [unwired: 1 in]
    }
    n129 = Array Max & Min(array=w216) -> (min value=w223:dbl)  [unwired: 3 out]
    n130 = Array Max & Min(array=w215) -> (min value=w221:dbl)  [unwired: 3 out]
    n131 = Array Max & Min(array=w214) -> (min value=w219:dbl)  [unwired: 3 out]
    n132 = Array Max & Min(array=w213) -> (min value=w217:dbl)  [unwired: 3 out]
    n133 = Array Max & Min(array=w181) -> (min value=w203:dbl)  [unwired: 3 out]
    n134 = Array Max & Min(array=w182) -> (min value=w201:dbl)  [unwired: 3 out]
    n135 = Array Max & Min(array=w183) -> (min value=w199:dbl)  [unwired: 3 out]
    n136 = Array Max & Min(array=w184) -> (min value=w197:dbl)  [unwired: 3 out]
    n137 = Array Max & Min(array=w185) -> (min value=w229:dbl)  [unwired: 3 out]
    n138 = Array Max & Min(array=w186) -> (min value=w198:dbl)  [unwired: 3 out]
    n139 = Array Max & Min(array=w187) -> (min value=w200:dbl)  [unwired: 3 out]
    n140 = Array Max & Min(array=w188) -> (min value=w202:dbl)  [unwired: 3 out]
    n141 = Array Max & Min(array=w194) -> (min value=w204:dbl)  [unwired: 3 out]
    n142 = Array Max & Min(array=w209) -> (min value=w218:dbl)  [unwired: 3 out]
    n143 = Array Max & Min(array=w210) -> (min value=w220:dbl)  [unwired: 3 out]
    n144 = Array Max & Min(array=w211) -> (min value=w222:dbl)  [unwired: 3 out]
    n145 = Array Max & Min(array=w212) -> (min value=w224:dbl)  [unwired: 3 out]
    n146 = Less?(x=w229, y=3000.0) -> (x < y?=w228:bool)
    n147 = Select(t=w229, s=w228, f=inf) -> (s? t:f=w230:dbl)
    n148 = Build Array(w230, w197, w198, w199, w200, w201, w202, w203, w204, w217, w218, w219, w220, w221, w222, w223, w224) -> (w196:dbl[])
    n149 = Array Max & Min(array=w196) -> (max value=w225:dbl, max index (indices)=w205:i32)  [unwired: 2 out]
    n150 = case shown="1" w205 {
      tunnel: [90.0 95.0 85.0 100.0 80.0 120.0 60.0 130.0 50.0 140.0 40.0 150.0 30.0 160.0 20.0 170.0 10.0] -> w206
      frame 0, Default {
      }
      frame 1 {
      }
      frame 2 {
      }
      frame 3 {
      }
      frame 4 {
      }
      frame 5 {
      }
      frame 6 {
      }
      frame 7 {
      }
      frame 8 {
      }
      frame 9 {
      }
      frame 10 {
      }
      frame 11 {
      }
      frame 12 {
      }
      frame 13 {
      }
      frame 14 {
      }
      frame 15 {
      }
      frame 16 {
      }
    }
    n151 = Less?(x=w225, y="length") -> (x < y?=→"VEstop":bool)
    n152 = Negate(x=w206) -> (-x=w207:dbl)
    n153 = Add(x=90.0, y=w207) -> (x+y=→"Anthena_Steer":dbl)
    n154 = expression code="(x/180.0)*pi" "degrees to radians"(w206) -> (w195:dbl)
    n155 = local read "Anthena_Steer"() -> (w160:i32)
    n156 = local read "TooClose"() -> (w158:bool)
    n157 = local read "NearSteer"() -> (w159:dbl)
    n158 = Polar To Re/Im(2:w195, 3:7000.0 ("r")) -> (0:w190:dbl, 1:w189:dbl)
    n159 = Build Array(w189, w175) -> (w191:dbl[])
    n160 = Build Array(w190, w175) -> (w192:dbl[])
    n161 = Select(t=w159, s=w158, f=w160) -> (s? t:f=→"inputsteer":dbl)
    n162 = Bundle(w191, w192) -> (→"TargetDerection":cluster{dbl[], dbl[]})  [unwired: 1 in]
    n163 = local read "Stop"() -> (w170:bool)
  }
  n164 = call-poly "VISA Configure Serial Port"("VISA resource name"="HENES", "timeout (10sec)"=u32 100, "Enable Termination\nChar (T)"=FALSE ("Enable Termination\nChar (T)"), "baud rate (9600)"=u32 115200) -> ("VISA resource name out"=w4:refnum<visa-resource-name>, "error out"=w3:errorcluster)  [unwired: 10 in]
  n165 = VISA Set I/O Buffer Size(VISA resource name=w4, mask (16)=w8, error in (no error)=w3) -> (VISA resource name out=w7:refnum<visa-resource-name>, error out=w6:errorcluster)  [unwired: 1 in]
  n166 = VISA Flush I/O Buffer(VISA resource name=w7, mask (16)=w5, error in (no error)=w6) -> (VISA resource name out=w17:refnum<visa-resource-name>, error out=w16:errorcluster)
  n167 = while {
    tunnel: w17 -> [w404]
    tunnel: w16 -> [w403]
    tunnel: [w397] -> w15
    tunnel: [w396] -> w14
    shift-right: [w391] -> _
    shift-left: w12 -> [w394]
    tunnel: w2 -> [w392]
    i -> [w398]
    stop <- w386 stop-if-true
    # "ERP_Racing Control"
    n168 = flat-sequence {
      tunnel: [w447] -> w401
      tunnel: [w446] -> w399
      tunnel: w404 -> [w449]
      tunnel: w403 -> [w448]
      tunnel: w398 -> [w445]
      tunnel: [w444] -> w395
      tunnel: w394 -> [w444]
      tunnel: w392 -> [w443]
      tunnel: [w453] -> w402
      tunnel: w401 -> [w453]
      tunnel: [w452] -> w400
      tunnel: w399 -> [w452]
      tunnel: w395 -> [w450]
      tunnel: [w450] -> w393
      tunnel: w402 -> [w481]
      tunnel: w400 -> [w480]
      tunnel: [w498] -> w397
      tunnel: [w497] -> w396
      tunnel: w393 -> [w472]
      tunnel: [w470] -> w391
      frame #0 {
        # "HENES RS232 프로토콜\nPC → 플랫폼"
        n169 = To Unsigned Byte Integer(number=w445) -> (unsigned 8bit integer=w434:u8)
        n170 = local read "inputsteer"() -> (w405:dbl)
        n171 = expression code="x*100"(w405) -> (w409:dbl)
        n172 = Boolean To (0,1)(Boolean="HLV_E-stop") -> (0, 1=w429:i16)
        n173 = Boolean To (0,1)(Boolean="HLV_A/M") -> (0, 1=w430:i16)
        n174 = To Word Integer(number=w409) -> (16bit integer=w412:i16)
        n175 = To Unsigned Byte Integer(number=w429) -> (unsigned 8bit integer=w427:u8)
        n176 = To Unsigned Byte Integer(number=w430) -> (unsigned 8bit integer=w428:u8)
        n177 = To Word Integer(number="InputSpeed") -> (16bit integer=w421:i16)
        n178 = In Range and Coerce(upper limit=i16 1999 ("상위 리미트"), x=w412, lower limit=i16 -1999 ("상위 리미트")) -> (coerced(x)=w420:i16)  [unwired: 1 out]
        n179 = Bundle By Name(cluster=w443, "HENES_M/A"=w428, "HENES_E-Stop"=w427, "HENES_Gear"="HLV_Gear 2", "HENES_Speed"=w421, "HENES_Steer"=w420, "HENES_Alive"=w434) -> (w436:T3)
        n180 = Unbundle By Name(w436) -> ("HENES_M/A"=w424:u8, "HENES_E-Stop"=w423:u8, "HENES_Gear"=w413:u8, "HENES_Speed"=w416:i16, "HENES_Steer"=w419:i16, "HENES_Alive"=w433:u8)
        n181 = Split Number(x=w419) -> (hi(x)=w418:u8, lo(x)=w417:u8)
        n182 = Split Number(x=w416) -> (hi(x)=w415:u8, lo(x)=w414:u8)
        n183 = Replace Array Subset(array=u8[] [83, 84, 88, 0, 0, 0, 0, 0, 0, 0, 0, 13, 10] ("unsigned byte array"), new element #1=w424, index #1=3, new element #2=w423, index #2=4, new element #3=w413, index #3=5, new element #4=w415, index #4=6, new element #5=w414, index #5=7, new element #6=w418, index #6=8, new element #7=w417, index #7=9, new element #8=w433, index #8=10) -> (w406:u8[])
        n184 = Byte Array To String(unsigned byte array=w406) -> (string=w408:string)
        "버퍼 쓰기" <- w408
        n185 = VISA Write(VISA resource name=w449, write buffer=w408, error in (no error)=w448) -> (VISA resource name out=w447:refnum<visa-resource-name>, error out=w446:errorcluster)  [unwired: 1 out]
      }
      frame #1 {
        n186 = Wait Until Next ms Multiple(millisecond multiple=u32 20 ("대기 시간 (ms)")) -> ()  [unwired: 1 out]
      }
      frame #2 {
        # "HENES RS232 프로토콜\n플랫폼 → PC"
        n187 = property class="Instr"(reference=w481, error in=w480) -> (reference out=w461:refnum<visa-resource-name>, error out=w460:errorcluster, "Serial Settings:Number of Bytes at Serial Port"=w459:u32)
        n188 = Greater?(x=w459, y=u32 14) -> (0:w477:bool)
        n189 = case shown="True" w477 {
          tunnel: w461 -> [w525 w530]
          tunnel: w460 -> [w524 w529]
          tunnel: [w525 w528] -> w479
          tunnel: [w524 w527] -> w478
          tunnel: w459 -> [_ w526]
          frame False {
          }
          frame True {
            n190 = VISA Read(VISA resource name=w530, byte count=w526, error in (no error)=w529) -> (VISA resource name out=w528:refnum<visa-resource-name>, error out=w527:errorcluster)  [unwired: 2 out]
          }
        }
        n191 = VISA Read(VISA resource name=w479, byte count=u32 13, error in (no error)=w478) -> (VISA resource name out=w498:refnum<visa-resource-name>, read buffer=w496:string, error out=w497:errorcluster)  [unwired: 1 out]
        "버퍼 읽기" <- w496
        n192 = Match Pattern(string=w496, regular expression="STX") -> (match substring=w493:string, after substring=w494:string)  [unwired: 1 in, 2 out]
        n193 = Concatenate Strings(w493, w494) -> (w492:string)
        n194 = String To Byte Array(string=w492) -> (unsigned byte array=w474:u8[])
        n195 = Index Array(array=w474, index #1=0, index #2=1, index #3=2) -> (element #1=w487:u8, element #2=w486:u8, element #3=w485:u8)
        n196 = Build Array(w487, w486, w485) -> (w484:u8[])
        n197 = Byte Array To String(unsigned byte array=w484) -> (string=w482:string)
        n198 = Equal?(x="STX", y=w482) -> (x = y?=w473:bool)
        n199 = case shown="True" w473 {
          tunnel: w474 -> [_ w523]
          tunnel: [w500 w510] -> w470
          tunnel: w472 -> [w500 w512]
          frame False {
          }
          frame True {
            n200 = Index Array(array=w523, index #1=3, index #2=4, index #3=5, index #4=6, index #5=7, index #6=8, index #7=9, index #8=10) -> (element #1=w511:u8, element #2=w509:u8, element #3=w508:u8, element #4=w507:u8, element #5=w506:u8, element #6=w504:u8, element #7=w503:u8, element #8=w501:u8)
            n201 = Join Numbers(hi=w507, lo=w506) -> ((hi.lo)=w514:u16)
            n202 = Join Numbers(hi=w504, lo=w503) -> ((hi.lo)=w513:u16)
            n203 = To Word Integer(number=w514) -> (16bit integer=w505:i16)
            n204 = To Word Integer(number=w513) -> (16bit integer=w502:i16)
            n205 = Bundle By Name(cluster=w512, "HLV_M/A_Status"=w511, "HLV_E-Stop"=w509, "HLV_Gear"=w508, "HLV_Speed"=w505, "HLV_Steer"=w502, "HLV_Alive"=w501) -> (w510:T6)
          }
        }
        n206 = Unbundle By Name(w470) -> ("HLV_M/A_Status"=w471:u8, "HLV_E-Stop"=w465:u8, "HLV_Gear"=→"Gear_Feed":u8, "HLV_Speed"=w463:i16, "HLV_Steer"=w462:i16, "HLV_Alive"=→"Alive_PCU":u8)
        n207 = To Double Precision Float(number=w463) -> (double precision float=w475:dbl)
        n208 = To Double Precision Float(number=w462) -> (double precision float=w468:dbl)
        n209 = Not Equal To 0?(x=w471) -> (x != 0?=→"Remote_M/A":bool)
        n210 = Not Equal To 0?(x=w465) -> (x != 0?=→"E-STOP":bool)
        n211 = expression code="x*0.01"(w475) -> (w454:dbl)
        "Speed_Feed(RPM)" <- w454
        n212 = expression code="x*0.01"(w468) -> (→"Steer_Feed":dbl)
        n213 = Divide(x=w454, y=60.0) -> (x/y=w458:dbl)
        n214 = Multiply(x=w458, y=0.848205) -> (x*y=→"Speed_Feed(m/s)":dbl)
      }
    }
    n215 = Tick Count (ms)() -> (millisecond timer value=w388:u32)
    n216 = feedback #3(u32 0 ("millisecond timer value")) -> (w389:u32)
    n217 = feedback-in #3(w388) -> ()
    n218 = Subtract(x=w388, y=w389) -> (x-y=→"HENES Loop Time":u32)
    n219 = local read "Stop"() -> (w386:bool)
  }
  n220 = flat-sequence {
    frame #0 {
      n221 = local write "InputSteer(cmd)"(0.0 ("InputSteer(cmd)")) -> ()
      n222 = Wait (ms)(milliseconds to wait=u32 1000) -> ()  [unwired: 1 out]
    }
    frame #1 {
      n223 = local write "HLV_Gear"(u8 2 ("HLV_Gear")) -> ()
    }
    frame #2 {
      n224 = while {
        stop <- w536 continue-if-true
        n225 = expression code="x/(0.00001*27*pi*60)"(6.0 ("Input_Spd(kph)")) -> (w539:dbl)
        n226 = local read "NearSteer"() -> (w534:dbl)
        n227 = Negate(x=w534) -> (-x=w535:dbl)
        n228 = expression code="x*4.35*1.8"(w539) -> (w537:dbl)
        n229 = local read "GoBack"() -> (w536:bool)
        n230 = local write "Input_Spd(cmd)"(w535) -> ()
        n231 = local write "Input_Spd(cmd)"(w537) -> ()
      }
    }
    frame #3 {
      w541 = 0.0 ("InputSteer(cmd)")
      n232 = Wait (ms)(milliseconds to wait=u32 1000) -> ()  [unwired: 1 out]
      n233 = local write "InputSteer(cmd)"(w541) -> ()
      n234 = local write "Input_Spd(cmd)"(w541) -> ()
    }
  }
  n235 = VISA Close(VISA resource name=w43, error in (no error)=w42) -> (error out=w44:errorcluster)
  n236 = call <vilib>:"Clear Errors.vi"("error in (no error)"=w44) -> ()  [unwired: 5 in, 2 out]
  n237 = while {
    stop <- w543 stop-if-true
    w546 = -450.0 ("element")
    w548 = 100.0 ("element")
    w547 = 450.0 ("element")
    w569 = 1200.0 ("f")
    w563 = 1200.0 ("element")
    w566 = 0.0 ("element")
    w570 = -300.0 ("element")
    w567 = 800.0 ("element")
    w571 = 100.0 ("element")
    w568 = 450.0 ("element")
    w560 = 0.0 ("element")
    w564 = -300.0 ("element")
    w561 = -800.0 ("element")
    w565 = 100.0 ("element")
    w562 = -450.0 ("element")
    # "뒤로 빠꾸"
    # "가까운 실제 존재 장애물은 피하기"
    # "Neer Steering"
    n238 = local read "X_arraysREAL"() -> (w545:i32[])
    n239 = local read "Y_arraysREAL"() -> (w544:i32[])
    n240 = local read "GoBack"() -> (w542:bool)
    n241 = Select(t=1700.0, s=w542, f=950.0 ("element")) -> (s? t:f=w559:dbl)
    n242 = Build Array(w562, w562, w561, w561, w560, w560, w562) -> (w585:dbl[])
    n243 = Build Array(w565, w564, w564, w563, w563, w565, w565) -> (w584:dbl[])
    n244 = Build Array(w568, w568, w567, w567, w566, w566, w568) -> (w577:dbl[])
    n245 = Build Array(w571, w570, w570, w569, w569, w571, w571) -> (w578:dbl[])
    n246 = Build Array(w547, w547, w546, w546, w547) -> (w556:dbl[])
    n247 = Build Array(w548, w559, w559, w548, w548) -> (w555:dbl[])
    n248 = call "ROI_IN_Check.vi"("도형Y좌표"=w584, "도형X좌표"=w585, "LiDAR_Y"=w544, "LiDAR_X"=w545) -> ("ROI_IN_Y"=w587:i32[], "ROI_IN_X"=w586:i32[])  [unwired: 6 in]
    n249 = Bundle(w585, w584) -> (→"NearCarROILeft":cluster{dbl[], dbl[]})  [unwired: 1 in]
    n250 = call "ROI_IN_Check.vi"("도형Y좌표"=w578, "도형X좌표"=w577, "LiDAR_Y"=w544, "LiDAR_X"=w545) -> ("ROI_IN_Y"=w590:i32[], "ROI_IN_X"=w589:i32[])  [unwired: 6 in]
    n251 = Bundle(w577, w578) -> (→"NearCarROIRight":cluster{dbl[], dbl[]})  [unwired: 1 in]
    n252 = call "ROI_IN_Check.vi"("도형Y좌표"=w555, "도형X좌표"=w556, "LiDAR_Y"=w544, "LiDAR_X"=w545) -> ("ROI_IN_Y"=w552:i32[], "ROI_IN_X"=w553:i32[])  [unwired: 6 in]
    n253 = Bundle(w556, w555) -> (→"GobackROI":cluster{dbl[], dbl[]})  [unwired: 1 in]
    n254 = Bundle("ROI_IN_X"=w586, "ROI_IN_Y"=w587) -> (→"NearCarPointsLeft":cluster{"ROI_IN_X":i32[], "ROI_IN_Y":i32[]})  [unwired: 1 in]
    n255 = Bundle("ROI_IN_X"=w589, "ROI_IN_Y"=w590) -> (→"NearCarPointsRight":cluster{"ROI_IN_X":i32[], "ROI_IN_Y":i32[]})  [unwired: 1 in]
    n256 = Re/Im To Polar(2:w587, 3:w586) -> (1:w588:dbl[])  [unwired: 1 out]
    n257 = Re/Im To Polar(2:w590, 3:w589) -> (1:w591:dbl[])  [unwired: 1 out]
    n258 = Re/Im To Polar(2:w552, 3:w553) -> (1:w551:dbl[])  [unwired: 1 out]
    n259 = Array Max & Min(array=w588) -> (min value=w592:dbl)  [unwired: 3 out]
    n260 = Array Size(array=w588) -> (size(s)=w583:i32)
    n261 = Array Max & Min(array=w591) -> (min value=w593:dbl)  [unwired: 3 out]
    n262 = Array Size(array=w591) -> (size(s)=w576:i32)
    n263 = Array Size(array=w551) -> (size(s)=w557:i32)
    n264 = Divide(x=40000.0, y=w592) -> (x/y=w595:dbl)
    n265 = Not Equal To 0?(x=w583) -> (x != 0?=w600:bool)
    n266 = Divide(x=-40000.0, y=w593) -> (x/y=w597:dbl)
    n267 = Not Equal To 0?(x=w576) -> (x != 0?=w599:bool)
    n268 = Not Equal To 0?(x=w557) -> (x != 0?=w558:bool)
    n269 = Select(t=w595, s=w600, f=0.0) -> (s? t:f=w596:dbl)
    n270 = Select(t=w597, s=w599, f=0.0) -> (s? t:f=w598:dbl)
    n271 = Or(x=w600, y=w599) -> (x .or. y?=→"TooClose":bool)
    n272 = Add(x=w596, y=w598) -> (x+y=→"NearSteer":dbl)
    n273 = local write "GoBack"(w558) -> ()
    n274 = local read "Stop"() -> (w543:bool)
  }
  n275 = VISA Flush I/O Buffer(VISA resource name=w15, error in (no error)=w14) -> (VISA resource name out=w18:refnum<visa-resource-name>, error out=w19:errorcluster)  [unwired: 1 in]
  n276 = VISA Close(VISA resource name=w18, error in (no error)=w19) -> (error out=w13:errorcluster)
  n277 = call <vilib>:"Simple Error Handler.vi"("error in (no error)"=w13) -> ()  [unwired: 4 in, 5 out]
  n278 = Close Python Session(session in=w28, error in=w29) -> (11:→"Clustering Error":errorcluster)
